vi "set_bit_depth.vi"(7 "calculate by timing? (F)":bool, 8 "error in (no error)":errorcluster, 10 "maximum bit-depth":i8, 11 "FPGAWrapperMH120124RAPS_PXI7813R in":refnum<class "FPGAWrapperMH120124RAPS_PXI7813R.lvclass">) -> (0 "error out":errorcluster, 3 "FPGAWrapperMH120124RAPS_PXI7813R out":refnum<class "FPGAWrapperMH120124RAPS_PXI7813R.lvclass">)   [LabVIEW 2010, in "FPGAWrapperMH120124RAPS_PXI7813R.lvclass"]
uses:
  FPGAWrapperMH120124RAPS_PXI7813R.lvclass
  FPGAWrapperMH120124RAPS_PXI7813R.lvclass/FPGAWrapperMH120124RAPS_PXI7813R.ctl
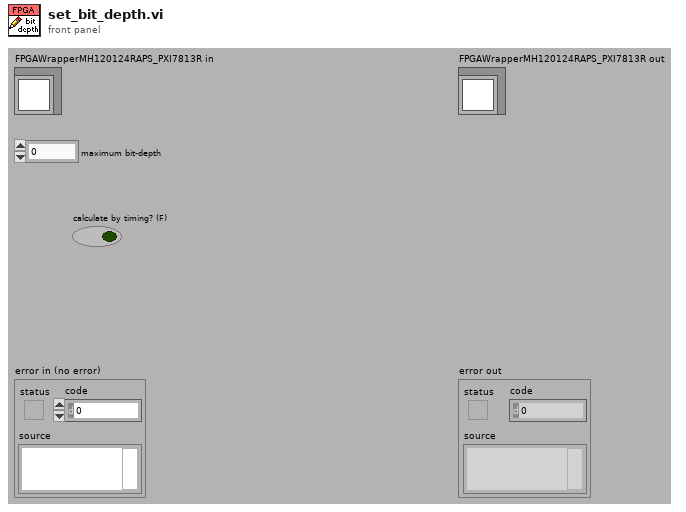
[diagram p1: front panel]
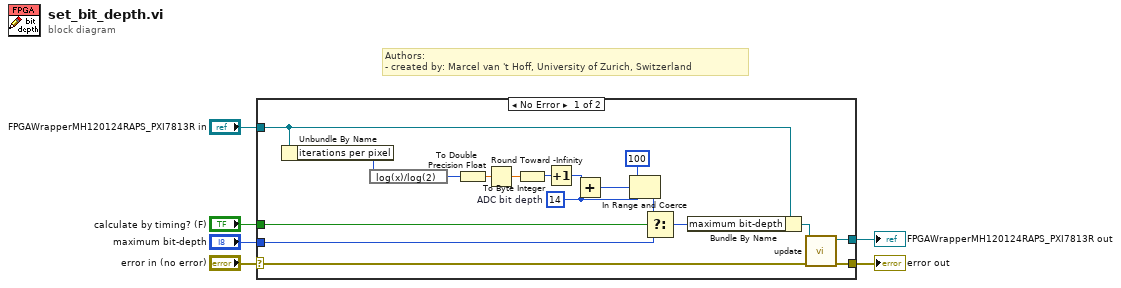
[diagram p0: block diagram]
diagram:
  # "Authors: \n- created by: Marcel van 't Hoff, University of Zurich, Switzerland"
  n1 = case shown="No Error" "error in (no error)" {
    selector: "error in (no error)" -> [w22 w25]
    tunnel: [w21 w25] -> w5
    tunnel: [w23 w26] -> w3
    tunnel: "FPGAWrapperMH120124RAPS_PXI7813R in" -> [w10 w26]
    tunnel: "maximum bit-depth" -> [w8 _]
    tunnel: "calculate by timing? (F)" -> [w11 _]
    frame No Error {
      w14 = i8 14  # ADC bit depth
      n2 = Unbundle By Name(w10) -> ("iterations per pixel"=w9:i32)
      n3 = expression code="log(x)/log(2)"(w9) -> (w19:i32)
      n4 = To Double Precision Float(number=w19) -> (double precision float=w17:dbl)
      n5 = Round Toward -Infinity(1:w17) -> (0:w18:dbl)
      n6 = To Byte Integer(number=w18) -> (8bit integer=w16:i8)
      n7 = Increment(x=w16) -> (x+1=w15:i8)
      n8 = Add(x=w15, y=w14) -> (x+y=w13:i8)
      n9 = In Range and Coerce(upper limit=i8 100, x=w13, lower limit=w14) -> (coerced(x)=w20:i8)  [unwired: 1 out]
      n10 = Select(t=w20, s=w11, f=w8) -> (s? t:f=w7:i8)
      n11 = Bundle By Name(cluster=w10, "maximum bit-depth"=w7) -> (w24:refnum<class "FPGAWrapperMH120124RAPS_PXI7813R.lvclass">)
      n12 = call-dynamic "update.vi"("error in (no error)"=w22, "FPGAWrapperMH120124RAPS_PXI7813R in"=w24) -> ("error out"=w21:errorcluster, "FPGAWrapperMH120124RAPS_PXI7813R out"=w23:refnum<class "FPGAWrapperMH120124RAPS_PXI7813R.lvclass">)  [unwired: 8 in]
    }
    frame Error {
    }
  }
  "error out" <- w5
  "FPGAWrapperMH120124RAPS_PXI7813R out" <- w3
